vi "Acquire Prompt Lock.vi"(8 "error in (no error)":errorcluster, 11 "GUI Element in":refnum<class "GUI Element.lvclass">) -> (0 "error out":errorcluster, 2 "Acquired":bool, 3 "GUI Element out":refnum<class "GUI Element.lvclass">)   [LabVIEW 2020, in "VolatusGUI.lvlib" / "GUI Element.lvclass"]
uses:
  GUI Element.lvclass
  GUI Element.lvclass/GUI Element.ctl
  lv-exec-anchor/ExecAnchor/ExecAnchor.lvclass
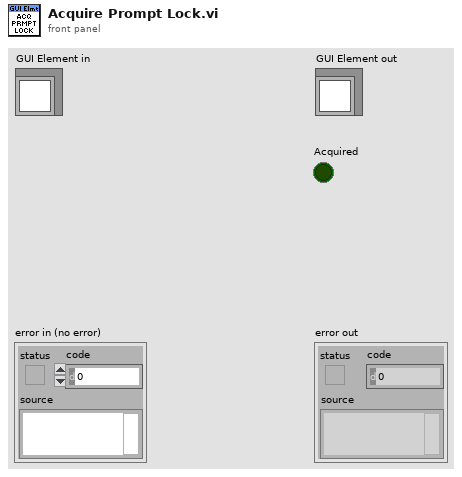
[diagram p1: front panel]
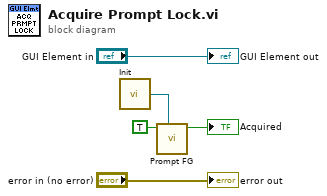
[diagram p0: block diagram]
diagram:
  n1 = call "Init.vi"() -> ("ExecAnchor out"=w1:refnum<class "ExecAnchor.lvclass">)  [unwired: 7 in]
  n2 = call "Prompt FG.vi"("ExecAnchor"=w1, "Set"=TRUE) -> ("Acquired"=→"Acquired":bool)  [unwired: 9 in]
  "error out" <- "error in (no error)"
  "GUI Element out" <- "GUI Element in"
